vi "Specialized Crossover.vi"(8 "error in (no error)":errorcluster, 9 "Parent 2":T1, 10 "Parent 1":T1, 11 "OSSP_Problem in":refnum<class "OSSP_Problem.lvclass">) -> (0 "error out":errorcluster, 1 "Child 2":T1, 2 "Child 1":T1, 3 "OSSP_Problem out":refnum<class "OSSP_Problem.lvclass">)   [LabVIEW 2013, in "GA.lvclass"]
uses:
  GA.lvclass
  Controls/Solution_GA.ctl
  OSSP_Problem.lvclass
  GanntChart.lvclass
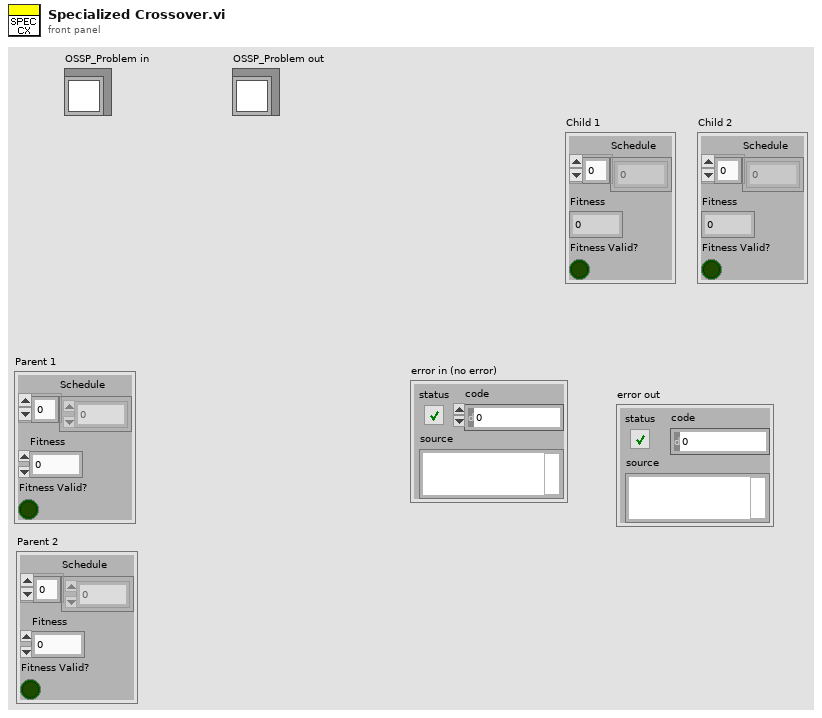
[diagram p1: front panel]
types:
  T1 = typedef "Solution_GA.ctl" = cluster{"Schedule":u16[], "Fitness":u16, "Fitness Valid?":bool}
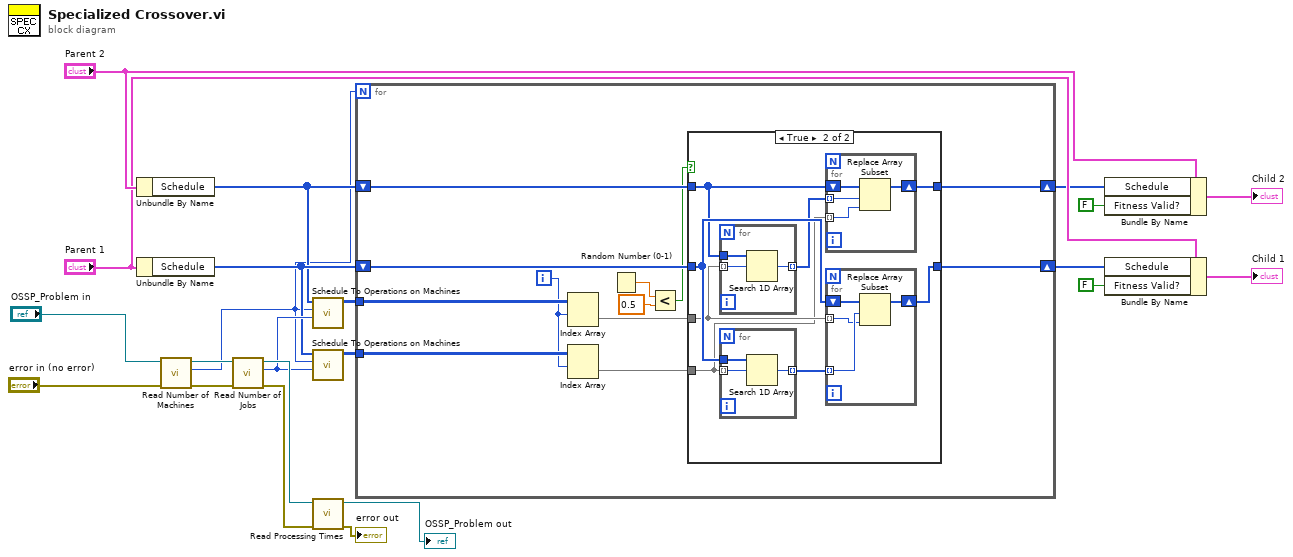
[diagram p0: block diagram]
diagram:
  n1 = Unbundle By Name("Parent 2") -> ("Schedule"=w6:u16[])
  n2 = Unbundle By Name("Parent 1") -> ("Schedule"=w7:u16[])
  n3 = call-dynamic "Read Number of Machines.vi"("error in (no error)"="error in (no error)", "OSSP_Problem in"="OSSP_Problem in") -> ("error out"=w16:errorcluster, "Number of Machines"=w3:i32, "OSSP_Problem out"=w14:refnum<class "OSSP_Problem.lvclass">)  [unwired: 7 in]
  n4 = call-dynamic "Read Number of Jobs.vi"("error in (no error)"=w16, "OSSP_Problem in"=w14) -> ("error out"=w15:errorcluster, "Number of Jobs"=w12:i32, "OSSP_Problem out"=w13:refnum<class "OSSP_Problem.lvclass">)  [unwired: 7 in]
  n5 = call "Schedule To Operations on Machines.vi"("Number of Jobs"=w12, "Number of Machines"=w3, "Schedule"=w6) -> ("Operations On Machines"=w5:i32[][])  [unwired: 8 in]
  n6 = call "Schedule To Operations on Machines.vi"("Number of Jobs"=w12, "Number of Machines"=w3, "Schedule"=w7) -> ("Operations On Machines"=w4:i32[][])  [unwired: 8 in]
  n7 = call-dynamic "Read Processing Times.vi"("error in (no error)"=w15, "OSSP_Problem in"=w13) -> ("error out"=→"error out":errorcluster, "OSSP_Problem out"=→"OSSP_Problem out":refnum<class "OSSP_Problem.lvclass">)  [unwired: 7 in, 1 out]
  n8 = for {
    N: w3 -> [_]
    tunnel: w4 -> [w28]
    tunnel: w5 -> [w30]
    shift-right: [w25] -> w2
    shift-left: w7 -> [w31]
    shift-right: [w24] -> w1
    shift-left: w6 -> [w32]
    i -> [w27]
    n9 = Index Array(array=w30, index (row)=w27) -> (element=w29:i32[])  [unwired: 1 in]
    n10 = Index Array(array=w28, index (row)=w27) -> (element=w26:i32[])  [unwired: 1 in]
    n11 = Random Number (0-1)() -> (number: 0 to 1=w33:dbl)
    n12 = Less?(x=w33, y=0.5) -> (x < y?=w23:bool)
    n13 = case shown="True" w23 {
      tunnel: w32 -> [w35 w40]
      tunnel: w31 -> [w36 w43]
      tunnel: w29 -> [_ w41]
      tunnel: w26 -> [_ w38]
      tunnel: [w36 w42] -> w25
      tunnel: [w35 w37] -> w24
      frame False {
      }
      frame True {
        n14 = for {
          tunnel: w41 -> [w51] mode=indexing
          tunnel: w40 -> [w50]
          tunnel: [w49] -> w39 mode=indexing
          n15 = Search 1D Array(1D array=w50, element=w51) -> (index of element=w49:i32)  [unwired: 1 in]
        }
        n16 = for {
          tunnel: w38 -> [w58] mode=indexing
          tunnel: w43 -> [w57]
          tunnel: [w56] -> w44 mode=indexing
          n17 = Search 1D Array(1D array=w57, element=w58) -> (index of element=w56:i32)  [unwired: 1 in]
        }
        n18 = for {
          tunnel: w39 -> [w47] mode=indexing
          tunnel: w38 -> [w46] mode=indexing
          shift-right: [w45] -> w37
          shift-left: w40 -> [w48]
          n19 = Replace Array Subset(array=w48, new element=w46, index=w47) -> (w45:u16[])
        }
        n20 = for {
          tunnel: w44 -> [w54] mode=indexing
          tunnel: w41 -> [w53] mode=indexing
          shift-right: [w52] -> w42
          shift-left: w43 -> [w55]
          n21 = Replace Array Subset(array=w55, new element=w53, index=w54) -> (w52:u16[])
        }
      }
    }
  }
  n22 = Bundle By Name(cluster="Parent 2", "Schedule"=w1, "Fitness Valid?"=FALSE) -> (→"Child 2":T1)
  n23 = Bundle By Name(cluster="Parent 1", "Schedule"=w2, "Fitness Valid?"=FALSE) -> (→"Child 1":T1)
